vi "setStopTime.vi"(8 "error in":errorcluster, 11 "TestRunner in":refnum<class "TestRunner.lvclass">) -> (0 "error out":errorcluster, 3 "TestRunner out":refnum<class "TestRunner.lvclass">)   [LabVIEW 2013, in "TestRunner.lvclass"]
uses:
  TestRunner.lvclass
  TestRunner.lvclass/TestRunner.ctl
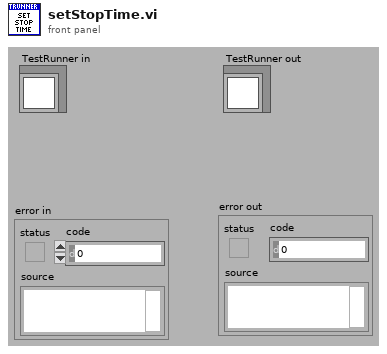
[diagram p1: front panel]
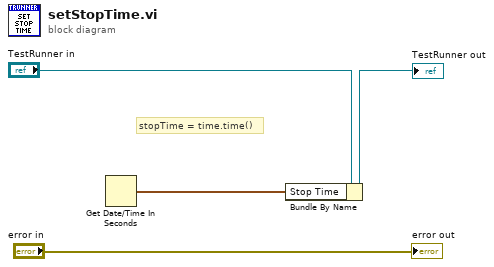
[diagram p0: block diagram]
diagram:
  # "stopTime = time.time()"
  n1 = Get Date/Time In Seconds() -> (seconds since 1Jan1904=w1:timestamp)
  n2 = Bundle By Name(cluster="TestRunner in", "Stop Time"=w1) -> (→"TestRunner out":refnum<class "TestRunner.lvclass">)
  "error out" <- "error in"
